vi "Tracker_v2_test_acq_comms_channel.vi"() -> ()   [LabVIEW 2016]
uses:
  <extravilib>/ChannelInstances/Stream-c(str,stamp)/Read With Abort.vi
  <extravilib>/ChannelInstances/Stream-c(str,stamp)/Endpoint.vi
  <extravilib>/ChannelInstances/Stream-c(str,stamp)/Instantiate.vi
  <extravilib>/ChannelInstances/Stream-c(str,stamp)/)Channel.vi
  <resource>/ChannelSupport/_ChannelSupport/WaitIfNeeded.vi
  <extravilib>/ChannelInstances/Stream-c(str,stamp).lvlib
panel:
  out "count":i32
  out "Instrument OK?":bool=TRUE
  out "Data frame channel sink":T1
  out "Data frame channel source":T2
  in  "Play/Pause":bool
  in  "Stop Button":bool
  in  "VISA resource name in":refnum<visa-resource-name>="ASRL3::INSTR"
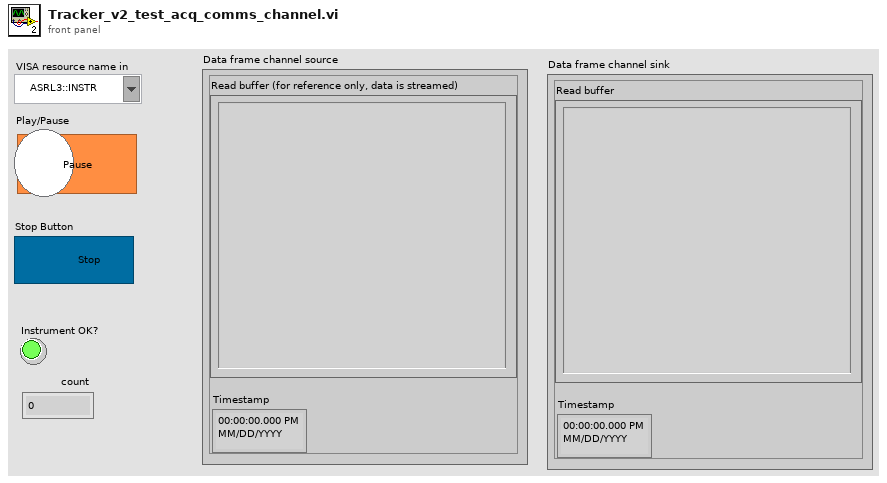
[diagram p1: front panel]
types:
  T1 = cluster{"Read buffer":string, "Timestamp":timestamp}
  T2 = cluster{"Read buffer (for reference only, data is streamed)":string, "Timestamp":timestamp}
  T3 = cluster{"Data acquisition status":refnum<notifier>, "Play/Pause status":refnum<notifier>, "Complete stop":refnum<notifier>, "Temp file ready for processing":refnum<notifier>, "Has been recorded":refnum<notifier>, "Recording now":refnum<notifier>, "Path to the latest complete temp file":refnum<notifier>, "Final CSV saved":refnum<notifier>, "Data loaded":refnum<notifier>}
  T4 = typedef "Stream-c(str,stamp).lvlib/)Channel.ctl" = refnum<queue>
  T5 = cluster{"Read buffer (for reference only, data is queued)":string, "Timestamp":timestamp}
  T6 = cluster{string, "seconds since 1Jan1904":timestamp}
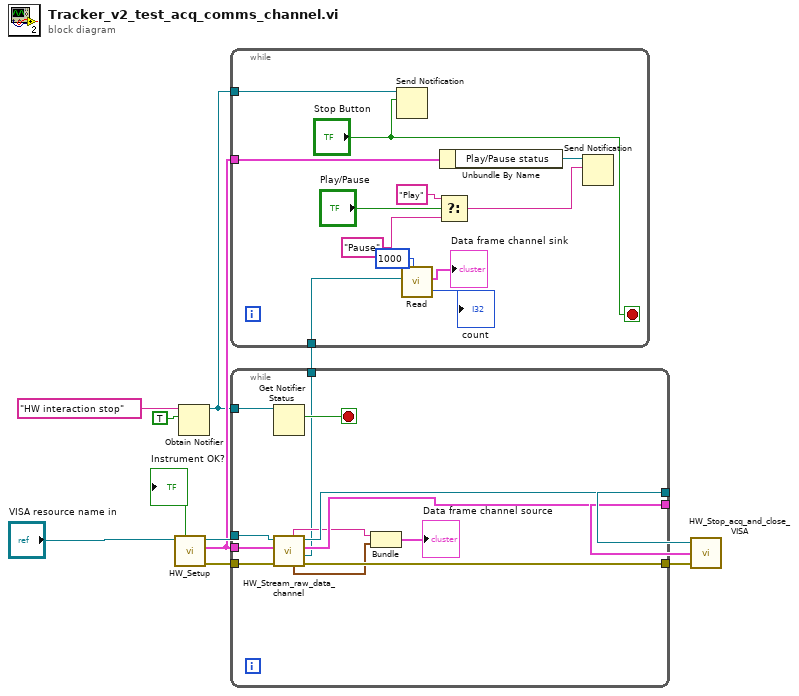
[diagram p0: block diagram]
diagram:
  n1 = call "HW_Setup.vi"("VISA resource name in"="VISA resource name in") -> ("VISA resource name out"=w11:refnum<visa-resource-name>, "Data flow controls"=w7:T3, "Instrument OK?"=→"Instrument OK?":bool, "error out"=w10:errorcluster)  [unwired: 3 in, 2 out]
  n2 = Obtain Notifier(name (unnamed)="HW interaction stop", notification data type=TRUE) -> (notifier out=w4:refnum<notifier>)  [unwired: 2 in, 2 out]
  n3 = while {
    tunnel: w11 -> [w24]
    tunnel: [w21] -> w9
    tunnel: w7 -> [w23]
    tunnel: [w20] -> w8
    tunnel: w10 -> [w22]
    tunnel: [w17] -> w3
    tunnel: w4 -> [w19]
    tunnel: [w13] -> w2
    stop <- w18 stop-if-true
    n4 = Get Notifier Status(notifier=w19) -> (current notification=w18:bool)  [unwired: 1 in, 4 out]
    n5 = call "HW_Stream_raw_data_channel.vi"("error in"=w22, "Data flow controls in"=w23, "VISA resource name in"=w24) -> ("error out"=w17:errorcluster, "Output data stream channel"=w13:T4, "Data flow controls out"=w20:T3, "VISA resource name out"=w21:refnum<visa-resource-name>, "Timestamp"=w15:timestamp, "Read buffer (for reference only, data is queued)"=w16:string)  [unwired: 3 in]
    n6 = Bundle("Read buffer (for reference only, data is queued)"=w16, "Timestamp"=w15) -> (→"Data frame channel source":T5)  [unwired: 1 in]
  }
  n7 = while {
    tunnel: w7 -> [w36]
    tunnel: w4 -> [w30]
    tunnel: w2 -> [w27]
    stop <- "Stop Button" stop-if-true
    n8 = Send Notification(notification="Stop Button", notifier=w30) -> ()  [unwired: 1 in, 2 out]
    n9 = call <extravilib>:"Read.vi"("timeout in ms (-1)"=1000, "channel"=w27) -> ("element"=→"Data frame channel sink":T6, "count"=→"count":i32)  [unwired: 5 in, 3 out]
    n10 = Select(t="Play", s="Play/Pause", f="Pause") -> (s? t:f=w33:string)
    n11 = Unbundle By Name(w36) -> ("Play/Pause status"=w35:refnum<notifier>)
    n12 = Send Notification(notification=w33, notifier=w35) -> ()  [unwired: 1 in, 2 out]
  }
  n13 = call "HW_Stop_acq_and_close_VISA.vi"("error in"=w3, "Data flow controls in"=w8, "VISA resource name in"=w9) -> ()  [unwired: 2 out]
